vi "Read URLs from Variant.vi"(8 "Error In":errorcluster, 9 "URL Section Data":variant, 10 "Channel Names":string[](array[string]), 11 "URL Prefix":string) -> (0 "Error Out":errorcluster, 2 "URLs":string[](array[string]), 3 "Found?":bool)   [LabVIEW 2013, in "CS++Utilities.lvlib"]
doc: "Read array of URL strings corresponding to specified Prefix and Channel Names from variant containing URL section data."
uses:
  CS++Utilities.lvlib
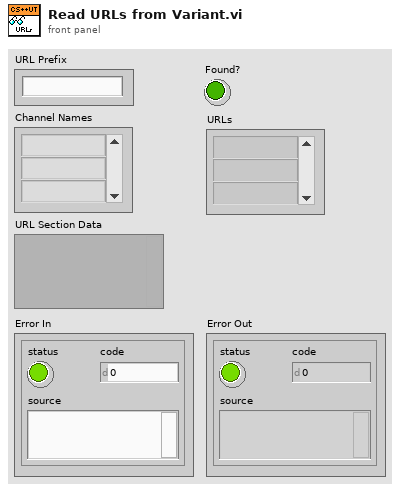
[diagram p1: front panel]
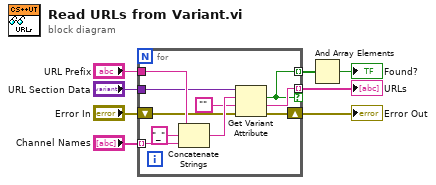
[diagram p0: block diagram]
diagram:
  n1 = for {
    tunnel: "Channel Names" -> [w17] mode=indexing
    tunnel: "URL Prefix" -> [w18]
    tunnel: "URL Section Data" -> [w16]
    shift-right: [w12] -> w1
    shift-left: "Error In" -> [w14]
    tunnel: [w10] -> w8 mode=indexing
    tunnel: [w11] -> w2 mode=indexing if=w10
    n2 = Concatenate Strings(w18, "_", w17) -> (w15:string)
    n3 = Get Variant Attribute(Variant=w16, name=w15, default value (empty Variant)="", error in=w14) -> (found=w10:bool, value=w11:string, error out=w12:errorcluster)  [unwired: 1 out]
  }
  "Error Out" <- w1
  "URLs" <- w2
  n4 = And Array Elements(Boolean array=w8) -> (logical AND=→"Found?":bool)
